vi "ITC503_T2n3Readout.vi"(0 "GPIB Address":i16, 3 "error in":errorcluster) -> (1 "Set T":string, 2 "error out":errorcluster, 4 "Sensor T1":string, 5 "Set T":dbl, 6 "Sensor T2":string, 7 "T2":dbl, 8 "T1":dbl, 9 "Sensor T3":string, 10 "T3":dbl)   [LabVIEW 2012]
uses:
  Oxford_itc503/BUSGEN.LLB/OxfordAddress.ctl
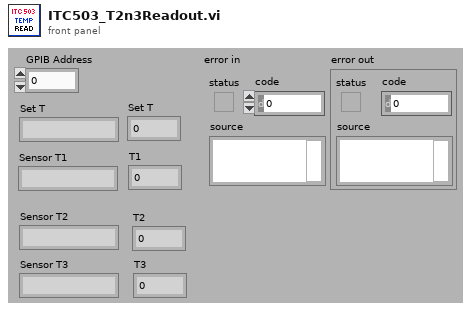
[diagram p1: front panel]
types:
  T1 = typedef "OxfordAddress.ctl" = cluster{"Com Port":i32, "ISOBUS Address":i32, "GPIB Address":i16, "Communication":enum16{"RS232", "ISOBUS", "GPIB", "Gateway"}}
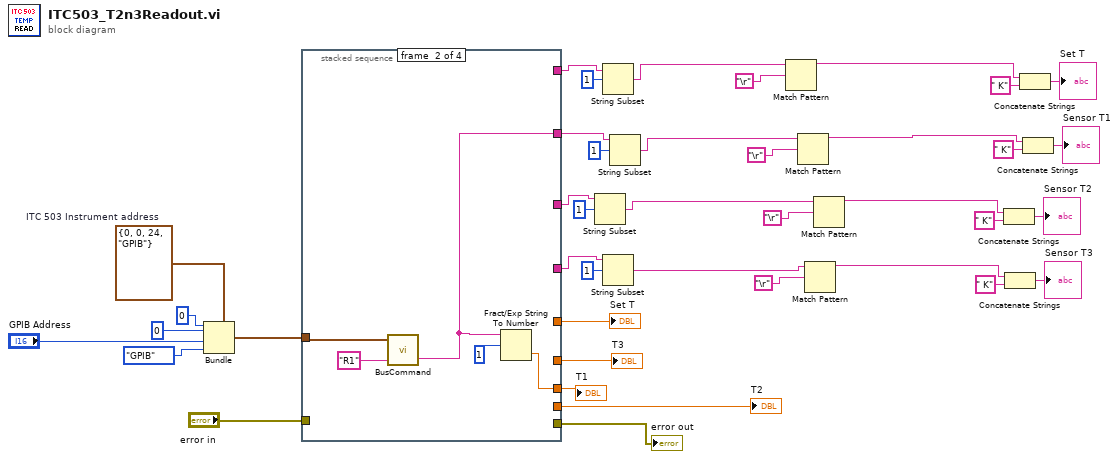
[diagram p0: block diagram]
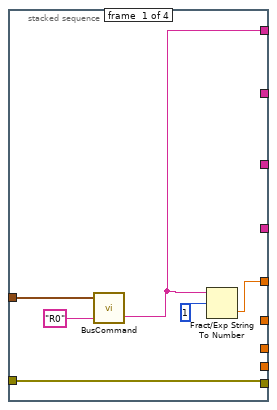
[diagram p2: hidden frame]
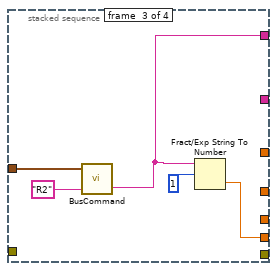
[diagram p3: hidden frame]
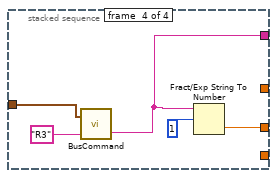
[diagram p4: hidden frame]
diagram:
  w38 = T1 {"Com Port"=0, "ISOBUS Address"=0, "GPIB Address"=24, "Communication"=enum."GPIB"}  # ITC 503 Instrument address
  n1 = Bundle(cluster=w38, "Com Port"=0, "ISOBUS Address"=0, "GPIB Address"="GPIB Address", "Communication"=enum16{"RS232", "ISOBUS", "GPIB", "Gateway"}."GPIB") -> (w33:T1)
  n2 = stacked-sequence {
    tunnel: [_ _ w54 _] -> w39
    tunnel: w33 -> [w43 w49 w53 w59]
    tunnel: [_ _ _ w58] -> w40
    tunnel: [_ _ _ w57] -> w13
    tunnel: [_ _ w52 _] -> w14
    tunnel: "error in" -> [w46 _ _ _]
    tunnel: [w46 _ _ _] -> w27
    tunnel: [w42 _ _ _] -> w16
    tunnel: [_ w48 _ _] -> w15
    tunnel: [w41 _ _ _] -> w24
    tunnel: [_ w47 _ _] -> w23
    frame #0 {
      n3 = call "BusCommand.vi"("Command"="R0", "Instrument address (in)"=w43) -> ("Reply"=w42:string)  [unwired: 1 out]
      n4 = Fract/Exp String To Number(string=w42, offset=1) -> (number=w41:dbl)  [unwired: 2 in, 1 out]
    }
    frame #1 {
      n5 = call "BusCommand.vi"("Command"="R1", "Instrument address (in)"=w49) -> ("Reply"=w48:string)  [unwired: 1 out]
      n6 = Fract/Exp String To Number(string=w48, offset=1) -> (number=w47:dbl)  [unwired: 2 in, 1 out]
    }
    frame #2 {
      n7 = call "BusCommand.vi"("Command"="R2", "Instrument address (in)"=w53) -> ("Reply"=w52:string)  [unwired: 1 out]
      n8 = Fract/Exp String To Number(string=w52, offset=1) -> (number=w54:dbl)  [unwired: 2 in, 1 out]
    }
    frame #3 {
      n9 = call "BusCommand.vi"("Command"="R3", "Instrument address (in)"=w59) -> ("Reply"=w57:string)  [unwired: 1 out]
      n10 = Fract/Exp String To Number(string=w57, offset=1) -> (number=w58:dbl)  [unwired: 2 in, 1 out]
    }
  }
  "T3" <- w40
  "T2" <- w39
  "error out" <- w27
  "Set T" <- w24
  "T1" <- w23
  n11 = String Subset(string=w14, offset (0)=1) -> (substring=w4:string)  [unwired: 1 in]
  n12 = String Subset(string=w16, offset (0)=1) -> (substring=w8:string)  [unwired: 1 in]
  n13 = String Subset(string=w13, offset (0)=1) -> (substring=w2:string)  [unwired: 1 in]
  n14 = String Subset(string=w15, offset (0)=1) -> (substring=w6:string)  [unwired: 1 in]
  n15 = Match Pattern(string=w8, regular expression="\r") -> (before substring=w7:string)  [unwired: 1 in, 3 out]
  n16 = Match Pattern(string=w6, regular expression="\r") -> (before substring=w5:string)  [unwired: 1 in, 3 out]
  n17 = Match Pattern(string=w2, regular expression="\r") -> (before substring=w1:string)  [unwired: 1 in, 3 out]
  n18 = Match Pattern(string=w4, regular expression="\r") -> (before substring=w3:string)  [unwired: 1 in, 3 out]
  n19 = Concatenate Strings(w3, " K" ("string")) -> (→"Sensor T2":string)
  n20 = Concatenate Strings(w1, " K" ("string")) -> (→"Sensor T3":string)
  n21 = Concatenate Strings(w7, " K" ("string")) -> (→"Set T":string)
  n22 = Concatenate Strings(w5, " K" ("string")) -> (→"Sensor T1":string)
